vi "2 Choose Set Point.vi"(10 "Assert Setpoint Array":bool[](array[boolean]), 11 "Setpoint Array":dbl[](array[numeric])) -> (3 "Setpoint":dbl)   [LabVIEW 2011]
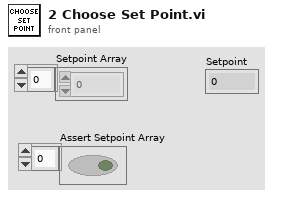
[diagram p1: front panel]
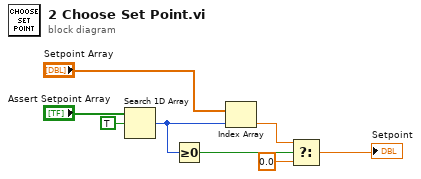
[diagram p0: block diagram]
diagram:
  n1 = Search 1D Array(1D array="Assert Setpoint Array", element=TRUE) -> (index of element=w4:i32)  [unwired: 1 in]
  n2 = Greater Or Equal To 0?(x=w4) -> (x >= 0?=w5:bool)
  n3 = Index Array(array="Setpoint Array", index=w4) -> (element=w3:dbl)
  n4 = Select(t=w3, s=w5, f=0.0) -> (s? t:f=→"Setpoint":dbl)
